vi "SetupDMA.vi"(0 "blocks":u32=1, 2 "Drv":u32=1, 3 "pixel":u32=2400, 4 "nos":u32=1) -> (1 "Data Values":u16[][](graph))   [LabVIEW 2017]
uses:
  ESLSCDLL.dll
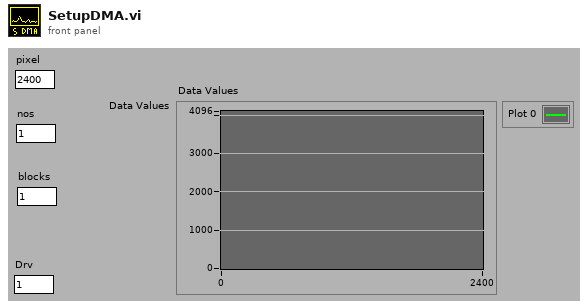
[diagram p1: front panel]
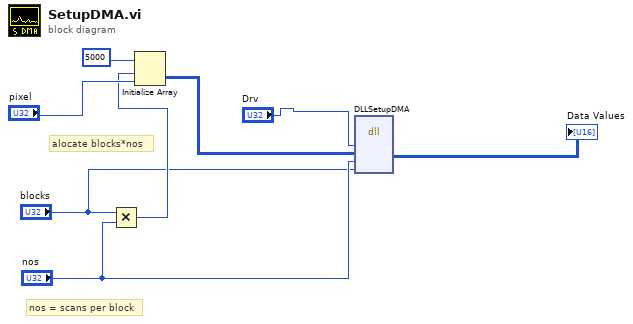
[diagram p0: block diagram]
diagram:
  # "alocate blocks*nos"
  # "nos = scans per block"
  n1 = Multiply(x="blocks", y="nos") -> (x*y=w3:u32)
  n2 = Initialize Array(u16 5000, w3, "pixel") -> (w7:u16[][])
  n3 = dll-call lib="C:/ENTW/PCIE/64bit/lv64/lv64/board.vis/ESLSCDLL.dll" fn="DLLSetupDMA" ("lwlscdll.dll:DLLReadFFLoop")("drv"="Drv", "dioden"=w7, "nos"="nos", "blocks"="blocks") -> ("dioden"=→"Data Values":u16[][])  [unwired: 7 in, 2 out]
